vi "Save Waveform.vi"(8 "error in (no error)":errorcluster, 11 "VISA resource name":refnum<visa-resource-name>) -> (0 "error out":errorcluster, 2 "Saved filename":string, 3 "VISA resource name out":refnum<visa-resource-name>)   [LabVIEW 2015, in "LeCroy Wave Series.lvlib"]
doc: "Saves the waveform as configured in the Save Waveform setup screen. Call the VI Configure Save Waveform.vi first."
uses:
  <instrlib>/LeCroy Wave Series/LeCroy Wave Series.lvlib
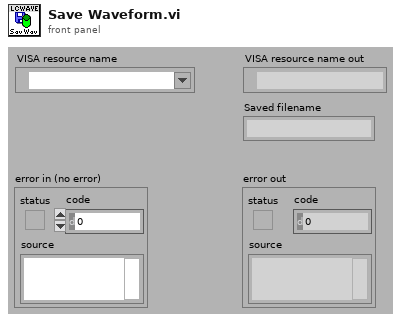
[diagram p1: front panel]
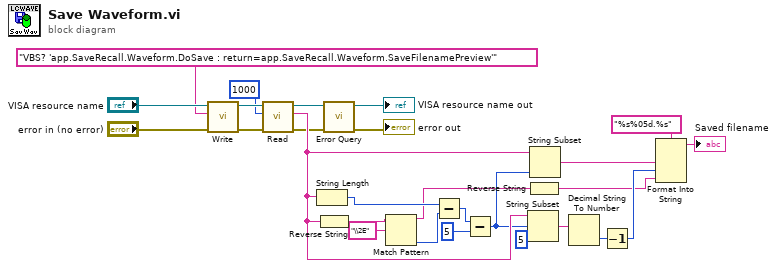
[diagram p0: block diagram]
diagram:
  n1 = call <instrlib>:"Write.vi"("error in (no error)"="error in (no error)", "Write Buffer"="VBS? 'app.SaveRecall.Waveform.DoSave : return=app.SaveRecall.Waveform.SaveFilenamePreview'", "VISA resource name"="VISA resource name") -> ("error out"=w23:errorcluster, "VISA resource name out"=w24:refnum<visa-resource-name>)  [unwired: 6 in, 1 out]
  n2 = call <instrlib>:"Read.vi"("error in (no error)"=w23, "Byte Count"=u32 1000, "VISA resource name"=w24) -> ("error out"=w3:errorcluster, "Read Buffer"=w12:string, "VISA resource name out"=w4:refnum<visa-resource-name>)  [unwired: 5 in, 1 out]
  n3 = String Length(string=w12) -> (length=w19:i32)
  n4 = Reverse String(1:w12) -> (0:w21:string)
  n5 = call <instrlib>:"Error Query.vi"("error in (no error)"=w3, "VISA resource name"=w4) -> ("error out"=→"error out":errorcluster, "VISA resource name out"=→"VISA resource name out":refnum<visa-resource-name>)  [unwired: 6 in, 2 out]
  n6 = Match Pattern(string=w21, regular expression="\\2E") -> (before substring=w10:string, offset past match=w18:i32)  [unwired: 1 in, 2 out]
  n7 = Subtract(x=w19, y=w18) -> (x-y=w17:i32)
  n8 = Subtract(x=w17, y=5) -> (x-y=w11:i32)
  n9 = String Subset(string=w12, offset (0)=w11, length (rest)=5 ("length (rest)")) -> (substring=w13:string)
  n10 = Reverse String(1:w10) -> (0:w6:string)
  n11 = String Subset(string=w12, length (rest)=w11) -> (substring=w7:string)  [unwired: 1 in]
  n12 = Decimal String To Number(string=w13) -> (number=w14:i32)  [unwired: 2 in, 1 out]
  n13 = Decrement(x=w14) -> (x-1=w8:i32)
  n14 = Format Into String(format string="%s%05d.%s", w7, w8, w6) -> (resulting string=→"Saved filename":string)  [unwired: 2 in, 1 out]
